vi "GetOneRecordFrom2DListCtrl.vi"(11 "testcaselist in":refnum<vi>) -> (2 "one record":string[](array[string]), 3 "testcaselist out":refnum<vi>)   [LabVIEW 2018, in "Library-Ctrl.lvlib"]
uses:
  Library-Ctrl.lvlib
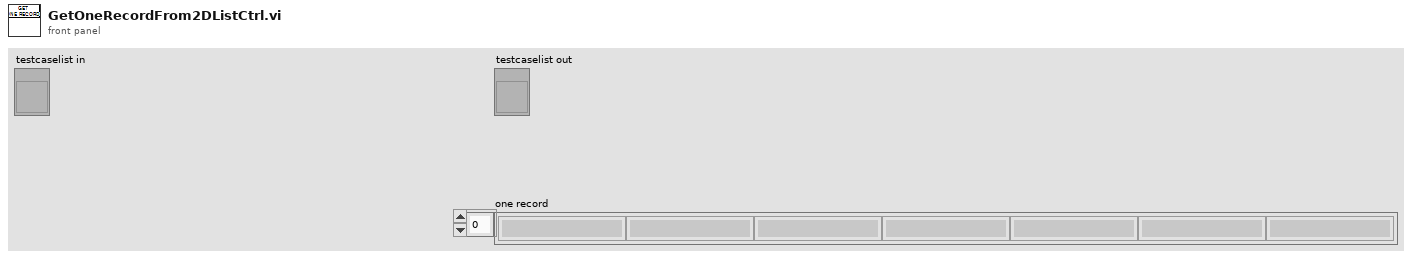
[diagram p1: front panel]
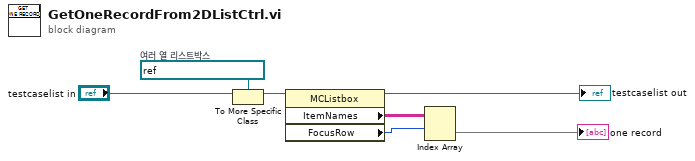
[diagram p0: block diagram]
diagram:
  w1 = refnum<vi> refnum  # 여러 열 리스트박스
  n1 = To More Specific Class(target class=w1, reference="testcaselist in") -> (specific class reference=w2:refnum<vi>)  [unwired: 1 in, 1 out]
  n2 = property class="MCListbox"(reference=w2) -> (reference out=→"testcaselist out":refnum<vi>, "ItemNames"=w7:string[][], "FocusRow"=w6:i32)  [unwired: 1 in, 1 out]
  n3 = Index Array(array=w7, index (row)=w6) -> (element=→"one record":string[])  [unwired: 1 in]
